vi "Close.vi"(8 "error in (no error)":errorcluster, 11 "Device in":refnum<class "Device.lvclass">) -> (0 "error out":errorcluster, 3 "Device out":refnum<class "Device.lvclass">)   [LabVIEW 2020, in "HAL.lvlib" / "Device.lvclass"]
uses:
  Device.lvclass
  Device State.ctl
  <vilib>/Utility/error.llb/Error Cluster From Error Code.vi
  <vilib>/ErrorRing/Error Ring.xnode
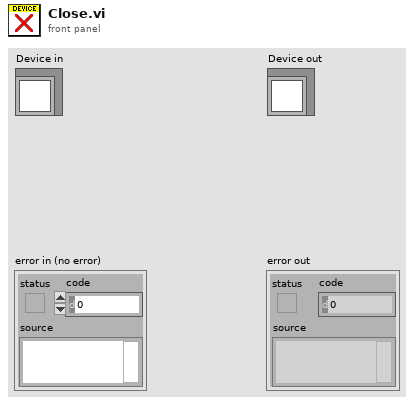
[diagram p1: front panel]
types:
  T1 = typedef "HAL.lvlib/Device.lvclass/Device State.ctl" = enum16{"Uninitialized", "Initialized", "Ready", "Running", "Error"}
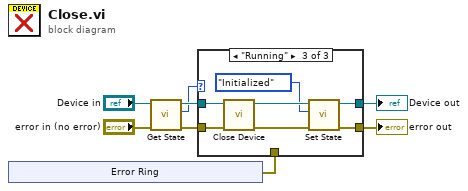
[diagram p0: block diagram]
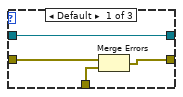
[diagram p2: hidden frame]
diagram:
  n1 = xnode "Error Ring"() -> ("error out"=w5:errorcluster)
  n2 = call "Get State.vi"("error in (no error)"="error in (no error)", "Device in"="Device in") -> ("error out"=w6:errorcluster, "Device State"=w7:T1, "Device out"=w8:refnum<class "Device.lvclass">)  [unwired: 7 in]
  n3 = case shown="\"Running\"" w7 {
    tunnel: w8 -> [w9 w14 w21]
    tunnel: w6 -> [w12 w13 w20]
    tunnel: [w9 w14 w16] -> w2
    tunnel: [w10 w13 w15] -> w3
    tunnel: w5 -> [w11 _ _]
    frame Default {
      n4 = Merge Errors(w12, w11) -> (w10:errorcluster)
    }
    frame "Initialized" {
    }
    frame "Running" {
      n5 = call-dynamic "Close Device.vi"("error in (no error)"=w20, "Device in"=w21) -> ("error out"=w17:errorcluster, "Device out"=w19:refnum<class "Device.lvclass">)  [unwired: 8 in]
      n6 = call "Set State.vi"("error in (no error)"=w17, "Device State"=Device_State."Initialized", "Device in"=w19) -> ("error out"=w15:errorcluster, "Device out"=w16:refnum<class "Device.lvclass">)  [unwired: 7 in]
    }
  }
  "error out" <- w3
  "Device out" <- w2
